vi "GetLatLong.vi"(11 "Fields":string[](array[string])) -> (1 "UTC Time Stamp":timestamp format="%<%.3X>T", 2 "Longitude":dbl format="%#_12f", 3 "Latitude":dbl format="%#_12f")   [LabVIEW 2024]
panel:
  # "Input"
  # "Output"
  # "$GNGGA,161632.000,5113.89332,N,00120.48498,W,1,06,2.1,70.1,M,47.2,M,,*6C"
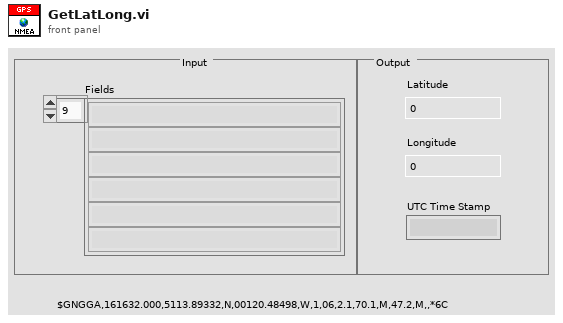
[diagram p1: front panel]
types:
  T1 = typedef "LVDateTimeRec.ctl" = cluster{"fractional second":dbl, "second":i32, "minute":i32, "hour":i32, "day of month":i32, "month":i32, "year":i32, "day of week":i32, "day of year":i32, "DST":i32}
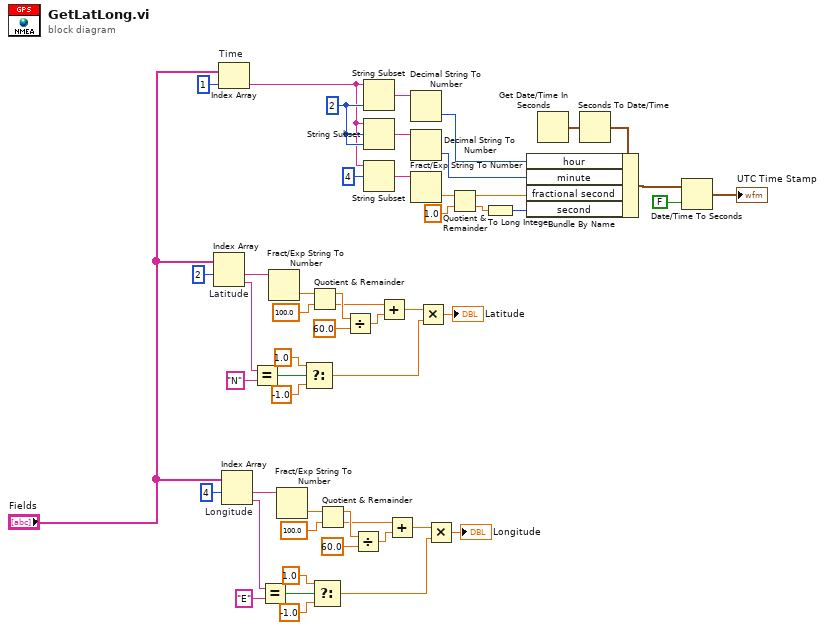
[diagram p0: block diagram]
diagram:
  w16 = 2 ("length (rest)")
  n1 = Index Array "Latitude"(array="Fields", index #1=2 ("index")) -> (element #1=w52:string, element #2=w45:string)  [unwired: 1 in]
  n2 = Index Array "Time"(array="Fields", index=1) -> (element=w4:string)
  n3 = Index Array "Longitude"(array="Fields", index #1=4 ("index")) -> (element #1=w23:string, element #2=w31:string)  [unwired: 1 in]
  n4 = Equal?(x=w45, y="N") -> (x = y?=w43:bool)
  n5 = Equal?(x=w31, y="E") -> (x = y?=w29:bool)
  n6 = Fract/Exp String To Number(string=w52) -> (number=w51:dbl)  [unwired: 3 in, 1 out]
  n7 = Fract/Exp String To Number(string=w23) -> (number=w37:dbl)  [unwired: 3 in, 1 out]
  n8 = Select(t=1.0, s=w43, f=-1.0 ("t")) -> (s? t:f=w39:dbl)
  n9 = Quotient & Remainder(x=w51, y=100.0) -> (x-y*floor(x/y)=w49:dbl, floor(x/y)=w47:dbl)
  n10 = Select(t=1.0, s=w29, f=-1.0 ("t")) -> (s? t:f=w25:dbl)
  n11 = Quotient & Remainder(x=w37, y=100.0) -> (x-y*floor(x/y)=w35:dbl, floor(x/y)=w33:dbl)
  n12 = Divide(x=w49, y=60.0) -> (x/y=w46:dbl)
  n13 = Divide(x=w35, y=60.0) -> (x/y=w32:dbl)
  n14 = String Subset(string=w4, length (rest)=w16) -> (substring=w12:string)  [unwired: 1 in]
  n15 = String Subset(string=w4, offset (0)=w16, length (rest)=w16) -> (substring=w13:string)
  n16 = String Subset(string=w4, offset (0)=4) -> (substring=w14:string)  [unwired: 1 in]
  n17 = Add(x=w47, y=w46) -> (x+y=w40:dbl)
  n18 = Add(x=w33, y=w32) -> (x+y=w26:dbl)
  n19 = Decimal String To Number(string=w12) -> (number=w5:i32)  [unwired: 2 in, 1 out]
  n20 = Decimal String To Number(string=w13) -> (number=w6:i32)  [unwired: 2 in, 1 out]
  n21 = Fract/Exp String To Number(string=w14) -> (number=w11:dbl)  [unwired: 3 in, 1 out]
  n22 = Multiply(x=w40, y=w39) -> (x*y=→"Latitude":dbl)
  n23 = Multiply(x=w26, y=w25) -> (x*y=→"Longitude":dbl)
  n24 = Quotient & Remainder(x=w11, y=1.0) -> (x-y*floor(x/y)=w9:dbl, floor(x/y)=w8:dbl)
  n25 = To Long Integer(number=w8) -> (32bit integer=w7:i32)
  n26 = Get Date/Time In Seconds() -> (seconds since 1Jan1904=w2:timestamp)
  n27 = Seconds To Date/Time(time stamp (now)=w2) -> (date time rec=w1:T1)  [unwired: 1 in]
  n28 = Bundle By Name(cluster=w1, "hour"=w5, "minute"=w6, "fractional second"=w9, "second"=w7) -> (w3:T1)
  n29 = Date/Time To Seconds(1:FALSE ("is UTC (F)"), 2:w3) -> (0:→"UTC Time Stamp":timestamp)
